vi "Software Update HCC Search And Index File Paths.vi"(8 "Error In":errorcluster, 11 "Newfi Exe Folder Path":path) -> (0 "Error Out":errorcluster, 2 "Index of File Path":i32[](array[numeric]), 3 "File Path":path[](array[path]))   [LabVIEW 2016]
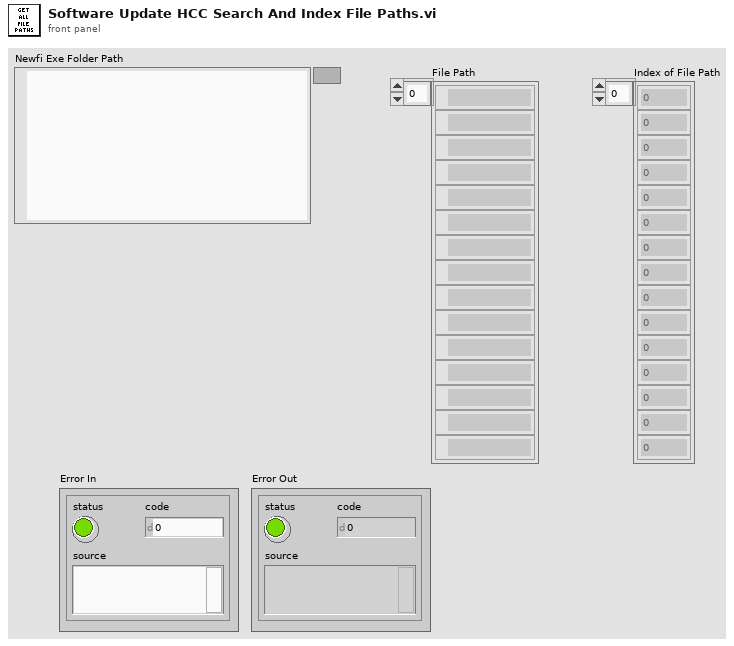
[diagram p1: front panel]
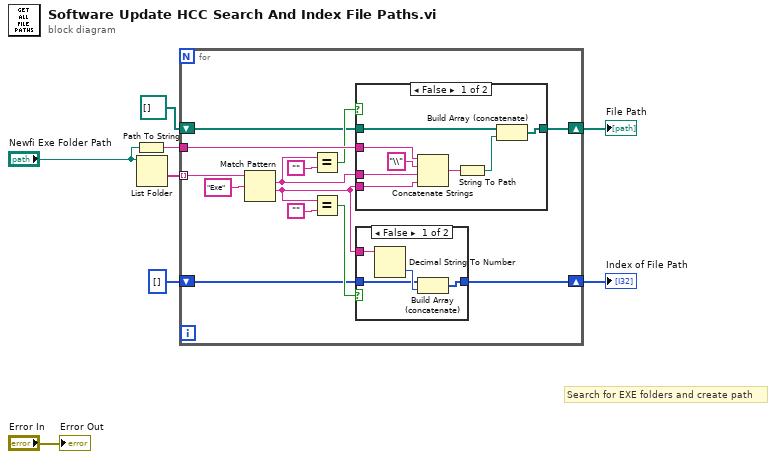
[diagram p0: block diagram]
diagram:
  # "Search for EXE folders and create path"
  n1 = Path To String(path="Newfi Exe Folder Path") -> (string=w8:string)
  n2 = List Folder(path="Newfi Exe Folder Path") -> (folder names=w7:string[])  [unwired: 3 in, 3 out]
  n3 = for {
    tunnel: w8 -> [w19]
    tunnel: w7 -> [w21] mode=indexing
    shift-right: [w14] -> w3
    shift-left: path[] [] -> [w15]
    shift-right: [w10] -> w4
    shift-left: i32[] [] -> [w11]
    n4 = Match Pattern(string=w21, regular expression="Exe") -> (match substring=w18:string, after substring=w9:string)  [unwired: 1 in, 2 out]
    n5 = Equal?(x=w18, y="") -> (x = y?=w16:bool)
    n6 = Equal?(x=w9, y="") -> (x = y?=w13:bool)
    n7 = case shown="False" w16 {
      tunnel: w19 -> [w34 _]
      tunnel: w18 -> [w33 _]
      tunnel: w9 -> [w32 _]
      tunnel: w15 -> [w30 w35]
      tunnel: [w29 w35] -> w14
      frame False {
        n8 = Concatenate Strings(w34, "\\" ("string"), w33, w32) -> (w28:string)
        n9 = String To Path(string=w28) -> (path=w27:path)
        n10 = Build Array (concatenate)(w30, w27) -> (w29:path[])
      }
      frame True {
      }
    }
    n11 = case shown="False" w13 {
      tunnel: w9 -> [w25 _]
      tunnel: w11 -> [w23 w26]
      tunnel: [w22 w26] -> w10
      frame False {
        n12 = Decimal String To Number(string=w25) -> (number=w24:i32)  [unwired: 2 in, 1 out]
        n13 = Build Array (concatenate)(w23, w24) -> (w22:i32[])
      }
      frame True {
      }
    }
  }
  "Index of File Path" <- w4
  "File Path" <- w3
  "Error Out" <- "Error In"
